vi "Write Cluster.vi"(8 "error in":errorcluster, 10 "Value Cluster in":variant, 11 "config-base in":refnum<class "config-base.lvclass">) -> (0 "error out":errorcluster, 3 "config-base out":refnum<class "config-base.lvclass">)   [LabVIEW 2022 SP3, in "hse-config.lvlib" / "config-base.lvclass"]
doc: "Set a cluster of config keys, can be nested. The cluster labels correspond to sections in the config-oject.\n\n____\nHAMPEL SOFTWARE ENGINEERING v3.8.0 (2023-12-18 14:41)"
uses:
  config-base.lvclass
  config-base.lvclass/config-base.ctl
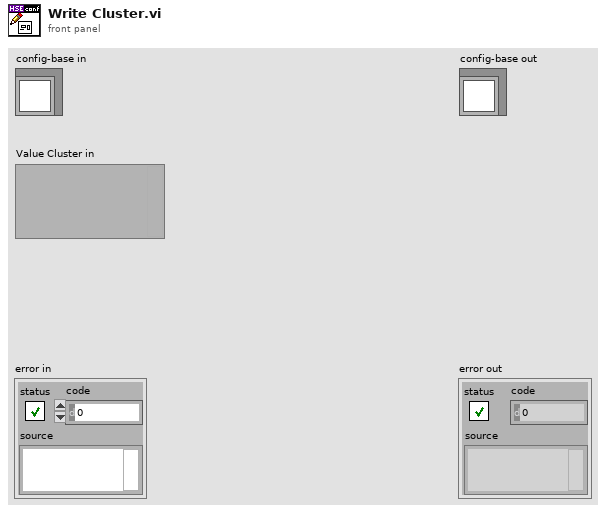
[diagram p1: front panel]
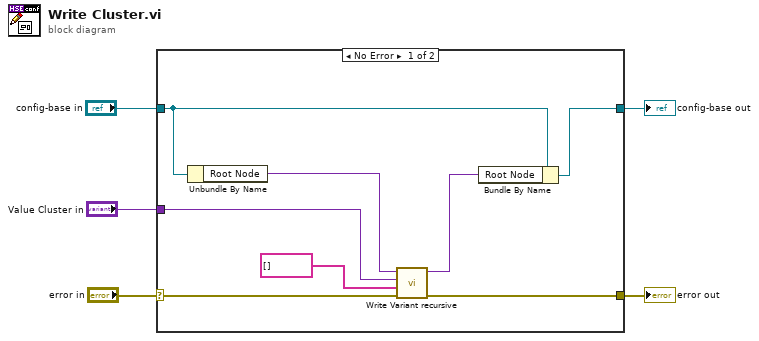
[diagram p0: block diagram]
diagram:
  n1 = case shown="No Error" "error in" {
    selector: "error in" -> [w13 w15]
    tunnel: [w7 w15] -> w4
    tunnel: [w9 w14] -> w2
    tunnel: "config-base in" -> [w11 w14]
    tunnel: "Value Cluster in" -> [w12 _]
    frame No Error {
      n2 = Unbundle By Name(w11) -> ("Root Node"=w10:variant)
      n3 = call "Write Variant recursive.vi"("error in (no error)"=w13, "Section"=string[] [], "Value Cluster in"=w12, "Root Node"=w10) -> ("error out"=w7:errorcluster, "Root Node out"=w8:variant)  [unwired: 6 in]
      n4 = Bundle By Name(cluster=w11, "Root Node"=w8) -> (w9:refnum<class "config-base.lvclass">)
    }
    frame Error {
    }
  }
  "error out" <- w4
  "config-base out" <- w2
